vi "_PC_Daemon_AO&DO.vi"(7 "eng_mode":refnum<vi>, 8 "error in (no error)":errorcluster) -> (0 "error out":errorcluster)   [LabVIEW 2018]
uses:
  <vilib>/event_ctls.llb/eventvkey.ctl
  RTFunc/_PC_RTFunc_AccessExtAO.vi
  RTFunc/_PC_RTFunc_AccessExtDI.vi
  RTFunc/_PC_RTFunc_AccessExtDO.vi
  PublicSubVI/Class/QMH/QMH.lvclass
panel:
  in  "Tab Control":T1(tab)
  in  "AO.Apply":bool
  in  "AO 7":cluster{"Label":string, "y":dbl}
  in  "AO 6":cluster{"Label":string, "y":dbl}
  in  "AO 5":cluster{"Label":string, "y":dbl}
  in  "AO 4":cluster{"Label":string, "y":dbl}
  in  "AO 3":cluster{"Label":string, "y":dbl}
  in  "AO 2":cluster{"Label":string, "y":dbl}
  in  "AO 1":cluster{"Label":string, "y":dbl}
  in  "AO 0":cluster{"Label":string, "y":dbl}
  in  "DO 7":cluster{"Label":string, "Boolean":bool}
  in  "DO 6":cluster{"Label":string, "Boolean":bool}
  in  "DO 5":cluster{"Label":string, "Boolean":bool}
  in  "DO 4":cluster{"Label":string, "Boolean":bool}
  in  "DO 3":cluster{"Label":string, "Boolean":bool}
  in  "DO 2":cluster{"Label":string, "Boolean":bool}
  in  "DO 1":cluster{"Label":string, "Boolean":bool}
  in  "DO 0":cluster{"Label":string, "Boolean":bool}
  in  "DO.Apply":bool
  in  "DI 7":cluster{"Label":string, "Boolean":bool}
  in  "DI 6":cluster{"Label":string, "Boolean":bool}
  in  "DI 5":cluster{"Label":string, "Boolean":bool}
  in  "DI 4":cluster{"Label":string, "Boolean":bool}
  in  "DI 3":cluster{"Label":string, "Boolean":bool}
  in  "DI 2":cluster{"Label":string, "Boolean":bool}
  in  "DI 1":cluster{"Label":string, "Boolean":bool}
  in  "DI 0":cluster{"Label":string, "Boolean":bool}
  in  "DI.Apply":bool
  out "stop":bool
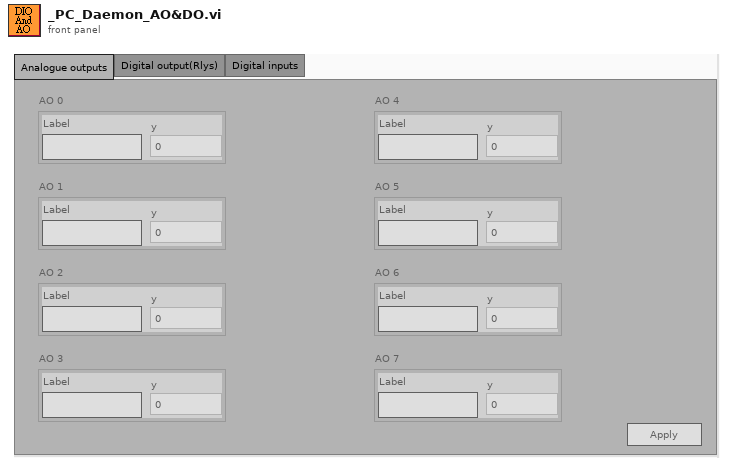
[diagram p1: front panel]
types:
  T1 = enum32{"Analogue outputs", "Digital output(Rlys)", "Digital inputs"}
  T2 = enum32{"Invalid", "Default", "Floating", "Floating/Auto-Hide", "Modal"}
  T3 = enum8{"Enabled", "Disabled", "Disabled and Grayed Out"}
  T4 = typedef "_ctl_RT_ExtAO.ctl" = cluster{"Label":string, "y":dbl}[]
  T5 = typedef "eventvkey.ctl" = enum16{"ASCII", "Enter", "Return", "Shift", "Ctrl", "Alt", "Cmd", "Opt", "Caps", "NumLock", "Clear", "Break", "Up", "Down", "Left", "Right", "Insert", "Delete", "Home", "End", "PageUp", "PageDown", "Escape", "Help", "Pause", "ScrollLock", "F1", "F2", "F3", "F4", "F5", "F6", "F7", "F8", "F9", "F10", "F11", "F12", "F13", "F14", "F15", "F16", "F17", "F18", "F19", "F20", "F21", "F22", "F23", "F24", "Play", "VolumeUp", "VolumeDown", "Mute", "Two Byte Char"}
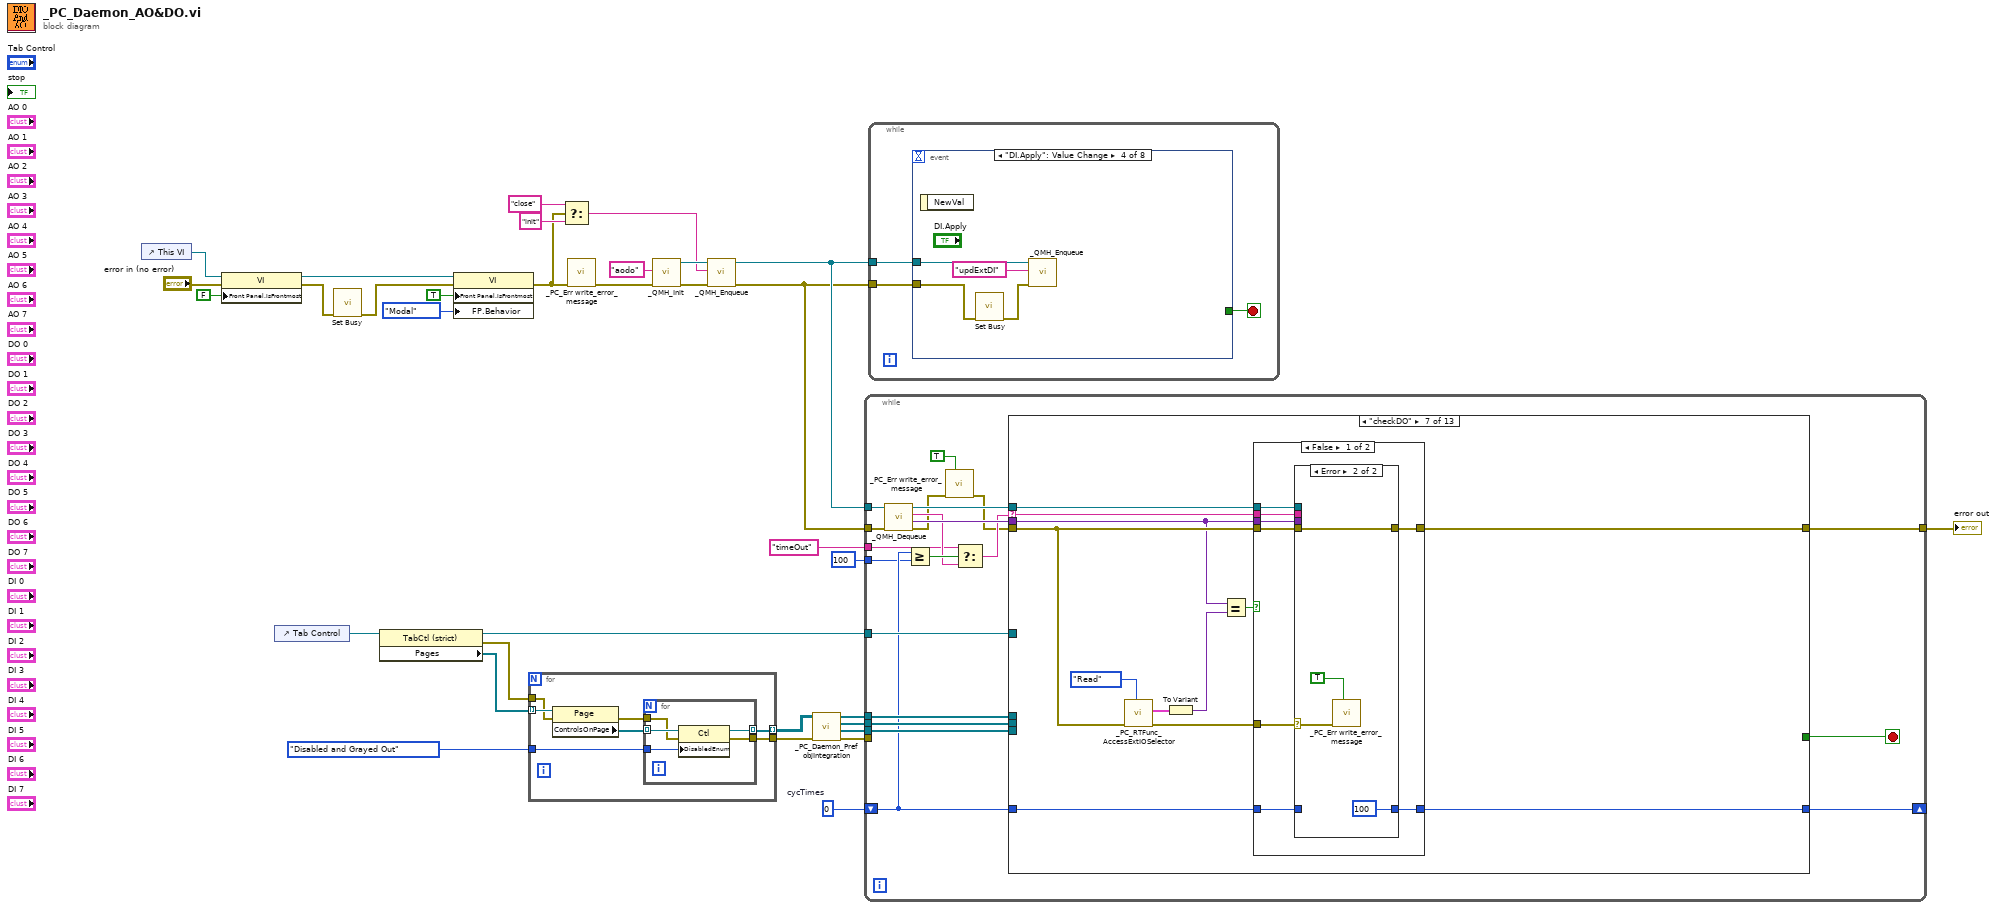
[diagram p0: block diagram]
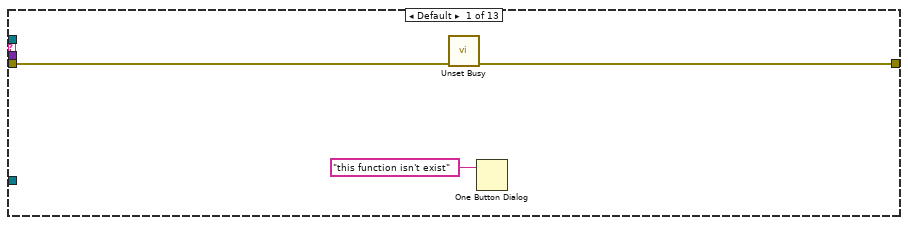
[diagram p2: hidden frame]
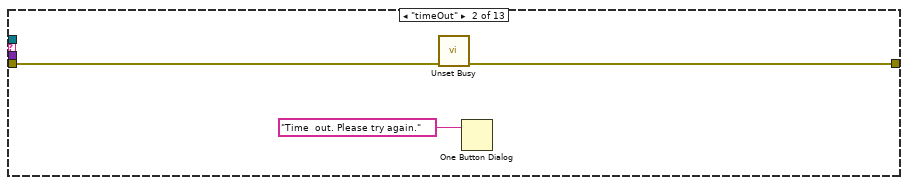
[diagram p3: hidden frame]
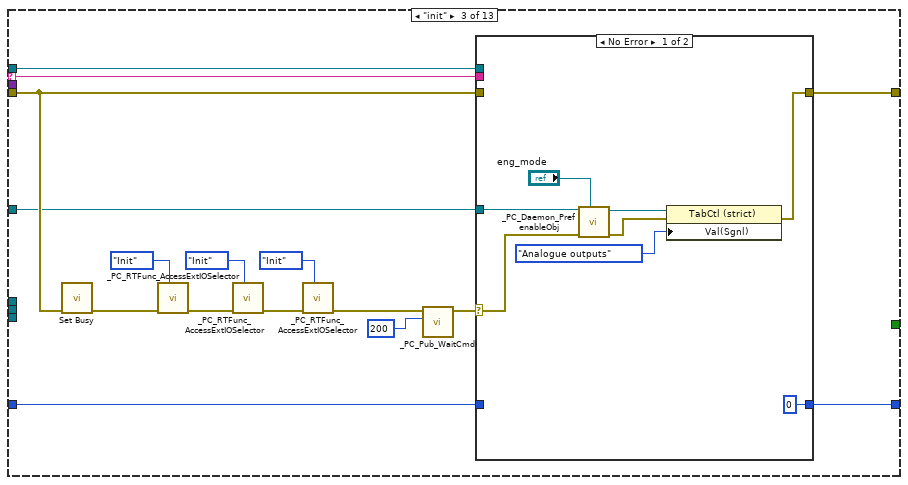
[diagram p4: hidden frame]
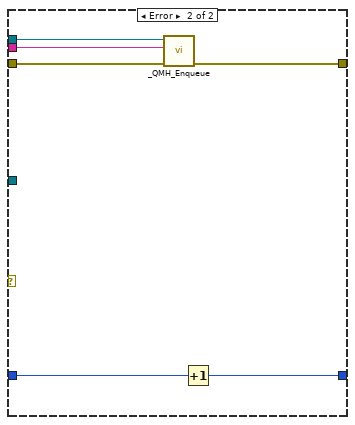
[diagram p5: hidden frame]
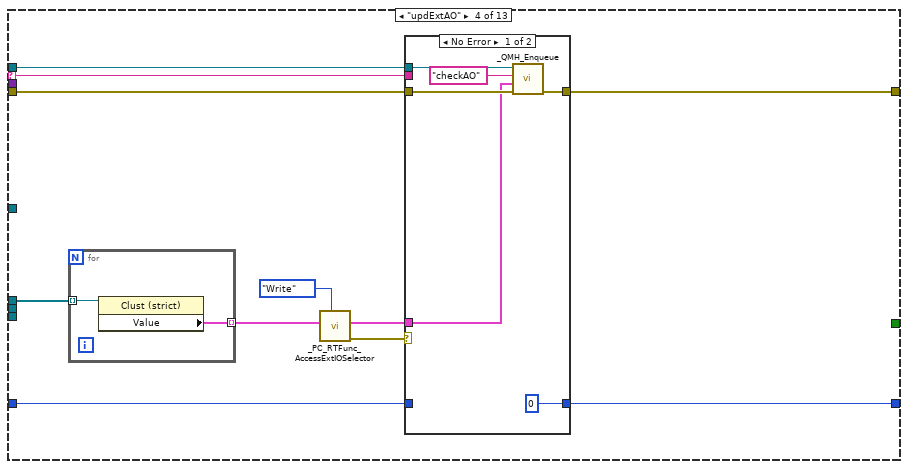
[diagram p6: hidden frame]
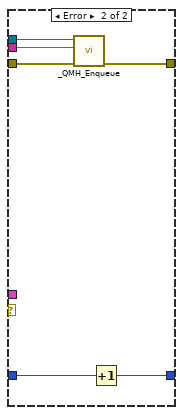
[diagram p7: hidden frame]
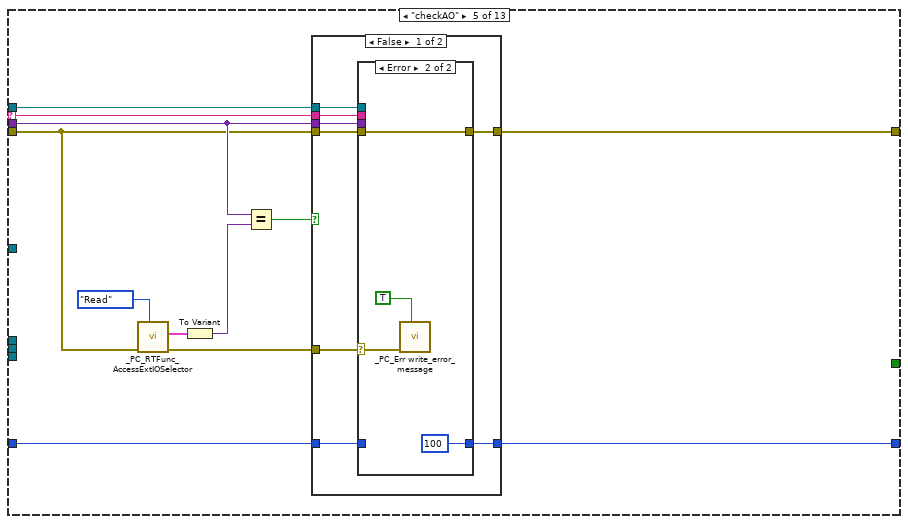
[diagram p8: hidden frame]
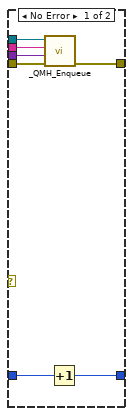
[diagram p9: hidden frame]
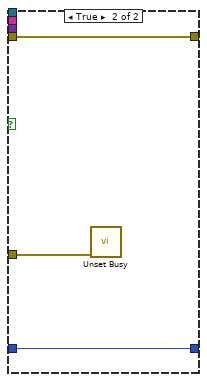
[diagram p10: hidden frame]
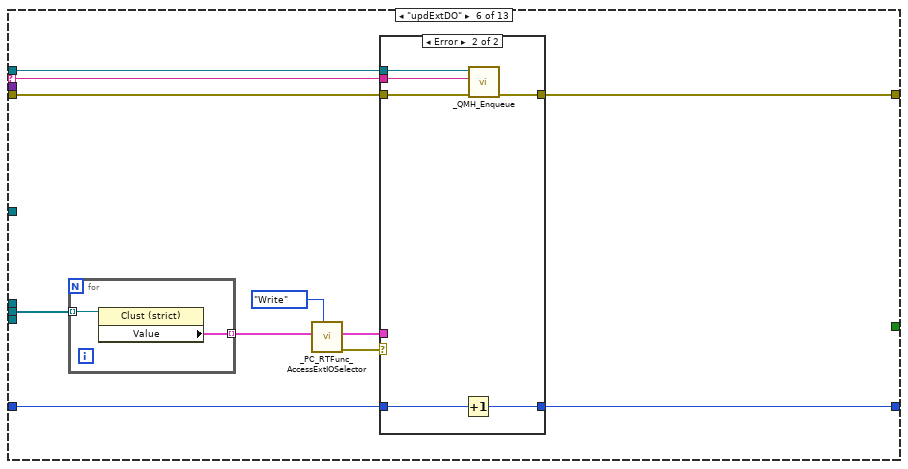
[diagram p11: hidden frame]
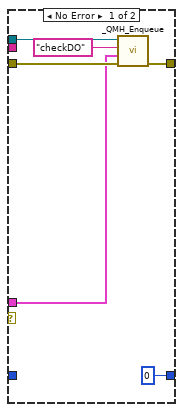
[diagram p12: hidden frame]
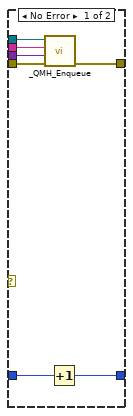
[diagram p13: hidden frame]
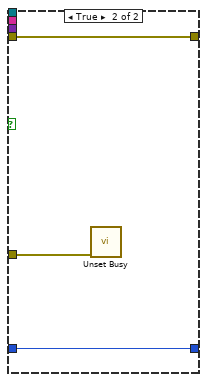
[diagram p14: hidden frame]
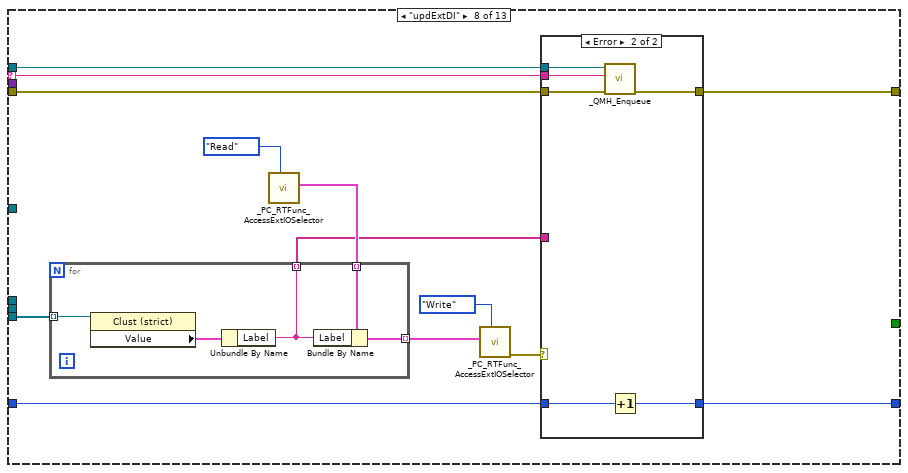
[diagram p15: hidden frame]
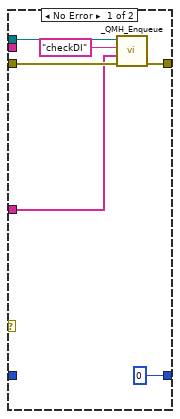
[diagram p16: hidden frame]
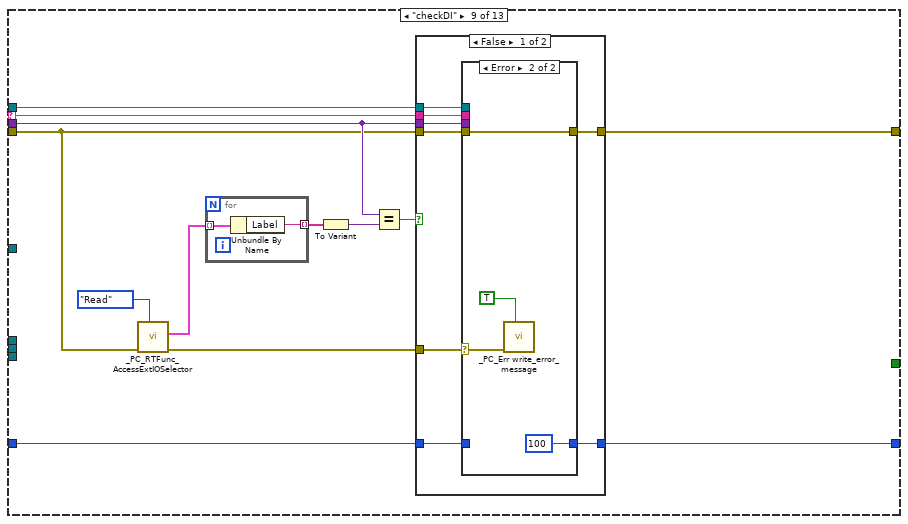
[diagram p17: hidden frame]
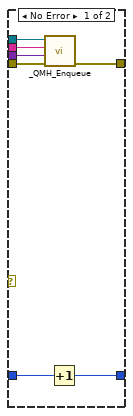
[diagram p18: hidden frame]
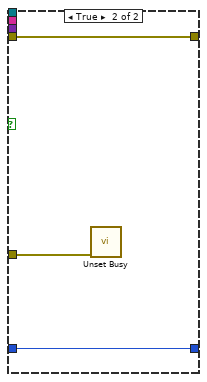
[diagram p19: hidden frame]
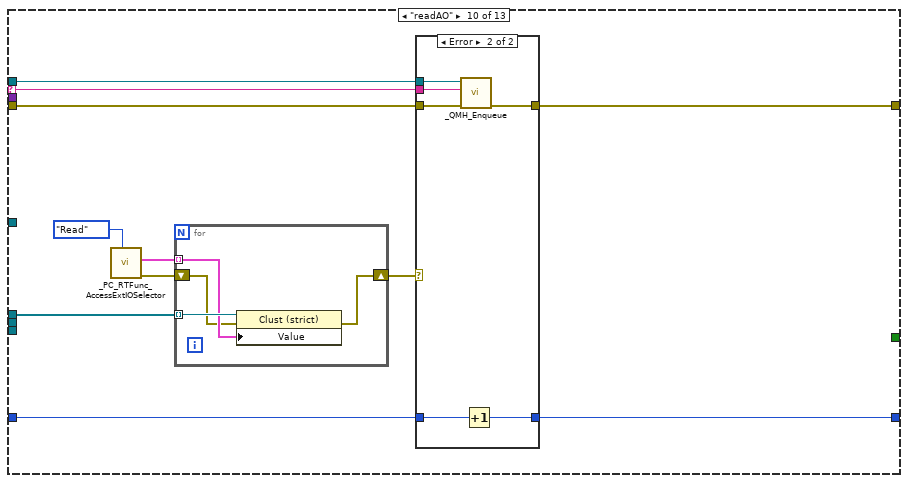
[diagram p20: hidden frame]
diagram:
  w3 = 0  # cycTimes
  n1 = control-ref of="This VI"() -> (w24:refnum<vi>)
  n2 = property class="VI"(reference=w24, error in="error in (no error)", "Front Panel.IsFrontmost"=FALSE) -> (reference out=w21:refnum<vi>, error out=w22:errorcluster)
  n3 = control-ref of="Tab Control"() -> (w33:refnum<vi>)
  n4 = call <vilib>:"Set Busy.vi"("error in (no error)"=w22) -> ("error out"=w20:errorcluster)  [unwired: 9 in, 1 out]
  n5 = property class="TabCtl (strict)"(reference=w33) -> (reference out=w5:refnum<vi>, error out=w32:errorcluster, "Pages"=w31:refnum<vi>[])  [unwired: 1 in]
  n6 = property class="VI"(reference=w21, error in=w20, "Front Panel.IsFrontmost"=TRUE ("Front Panel Window:Is Frontmost"), "FP.Behavior"=T2."Modal" ("Front Panel Window:Behavior")) -> (error out=w13:errorcluster)  [unwired: 1 out]
  n7 = for {
    tunnel: w31 -> [w40] mode=indexing
    tunnel: T3."Disabled and Grayed Out" ("Disabled") -> [w39]
    tunnel: [w37] -> w28
    tunnel: w32 -> [w35]
    tunnel: [w34] -> w29 mode=indexing
    n8 = property class="Page"(reference=w40, error in=w35) -> (error out=w36:errorcluster, "ControlsOnPage"=w38:refnum<vi>[])  [unwired: 1 out]
    n9 = for {
      tunnel: w38 -> [w45] mode=indexing
      tunnel: w39 -> [w44]
      tunnel: [w43] -> w37
      tunnel: w36 -> [w42]
      tunnel: [w41] -> w34 mode=indexing
      n10 = property class="Ctl"(reference=w45, error in=w42, "DisabledEnum"=w44) -> (reference out=w41:refnum<vi>, error out=w43:errorcluster)
    }
  }
  n11 = Select(t="close" ("name (unnamed)"), s=w13, f="init") -> (s? t:f=w15:string)
  n12 = call "_PC_Err write_error_message.vi"("error in"=w13) -> ("error out"=w12:errorcluster)  [unwired: 10 in]
  n13 = call "_QMH_Init.vi"("error in (no error)"=w12, "name (unnamed)"="aodo") -> ("error out"=w14:errorcluster, "QMH out"=w16:refnum<class "QMH.lvclass">)  [unwired: 8 in]
  n14 = call "_QMH_Enqueue.vi"("error in (no error)"=w14, "Msg"=w15, "QMH in"=w16) -> ("error out"=w10:errorcluster, "QMH out"=w11:refnum<class "QMH.lvclass">)  [unwired: 7 in]
  n15 = call "_PC_Daemon_Pref objIntegration.vi"("error in (no error)"=w28, "tabObjRefnum"=w29) -> ("error out"=w6:errorcluster, "DI"=w7:refnum<vi>[], "DO"=w8:refnum<vi>[], "AO"=w9:refnum<vi>[])  [unwired: 6 in]
  n16 = while {
    tunnel: w9 -> [w63]
    tunnel: w11 -> [w65]
    tunnel: w10 -> [w64]
    tunnel: w5 -> [w60]
    tunnel: w8 -> [w59]
    tunnel: w7 -> [w58]
    tunnel: w6 -> [_]
    tunnel: [w56] -> w4
    shift-right: [w55] -> _
    shift-left: w3 -> [w54]
    tunnel: 100 ("y") -> [w53]
    tunnel: "timeOut" ("t") -> [w49]
    stop <- w57 stop-if-true
    n17 = call "_QMH_Dequeue.vi"("error in (no error)"=w64, "QMH in"=w65) -> ("error out"=w47:errorcluster, "Data"=w61:variant, "Msg"=w51:string, "QMH out"=w62:refnum<class "QMH.lvclass">)  [unwired: 4 in, 2 out]
    n18 = Greater Or Equal?(x=w54, y=w53) -> (x >= y?=w52:bool)
    n19 = call "_PC_Err write_error_message.vi"("show msg( T )"=TRUE, "error in"=w47) -> ("error out"=w46:errorcluster)  [unwired: 9 in]
    n20 = Select(t=w49, s=w52, f=w51) -> (s? t:f=w50:string)
    n21 = case shown="\"checkDO\"" w50 {
      selector: w50 -> [_ _ w75 w107 w131 w166 w190 w228 w257 w291 w316 w340 _]
      tunnel: w63 -> [_ _ _ w106 _ _ _ _ _ w295 _ _ _]
      tunnel: w46 -> [w67 w70 w77 w108 w129 w167 w191 w229 w255 w290 w315 w339 w360]
      tunnel: w62 -> [_ _ w78 w109 w132 w168 w192 w230 w258 w292 w317 w341 w361]
      tunnel: w61 -> [_ _ _ _ w130 _ w189 _ w256 _ _ _ _]
      tunnel: w60 -> [_ _ w76 _ _ _ _ _ _ _ _ _ _]
      tunnel: w59 -> [_ _ _ _ _ w164 _ _ _ _ w318 _ _]
      tunnel: w58 -> [_ _ _ _ _ _ _ w226 _ _ _ w342 _]
      tunnel: [_ _ _ _ _ _ _ _ _ _ _ _ TRUE] -> w57
      tunnel: [w66 w69 w72 w102 w128 w161 w186 w220 w250 w287 w314 w335 w359] -> w56
      tunnel: w54 -> [_ _ w74 w104 w135 w163 w188 w222 w252 w289 w312 w337 _]
      tunnel: [_ _ w73 w103 w127 w162 w187 w221 w251 w288 w313 w336 _] -> w55
      frame Default {
        n22 = call <vilib>:"Unset Busy.vi"("error in (no error)"=w67) -> ("error out"=w66:errorcluster)  [unwired: 10 in]
        n23 = One Button Dialog(message="this function isn't exist") -> ()  [unwired: 1 in, 1 out]
      }
      frame "timeOut" {
        n24 = call <vilib>:"Unset Busy.vi"("error in (no error)"=w70) -> ("error out"=w69:errorcluster)  [unwired: 10 in]
        n25 = One Button Dialog(message="Time  out. Please try again.") -> ()  [unwired: 1 in, 1 out]
      }
      frame "init" {
        n26 = call <vilib>:"Set Busy.vi"("error in (no error)"=w77) -> ("error out"=w82:errorcluster)  [unwired: 9 in, 1 out]
        n27 = call-poly "_PC_RTFunc_AccessExtIOSelector.vi"("Function"=enum16{"Init", "Write", "Read"}."Init", "error in (no error)"=w82) -> ("error out"=w84:errorcluster)  [unwired: 8 in, 1 out]
        n28 = call-poly "_PC_RTFunc_AccessExtIOSelector.vi"("Function"=enum16{"Init", "Write", "Read"}."Init", "error in (no error)"=w84) -> ("error out"=w83:errorcluster)  [unwired: 8 in, 1 out]
        n29 = call-poly "_PC_RTFunc_AccessExtIOSelector.vi"("Function"=enum16{"Init", "Write", "Read"}."Init", "error in (no error)"=w83) -> ("error out"=w80:errorcluster)  [unwired: 8 in, 1 out]
        n30 = call "_PC_Pub_WaitCmd.vi"("milliseconds to wait"=u32 200, "error in (no error)"=w80) -> ("error out"=w79:errorcluster)  [unwired: 9 in]
        n31 = case shown="No Error" w79 {
          selector: w79 -> [w93 _]
          tunnel: w78 -> [_ w101]
          tunnel: w77 -> [_ w100]
          tunnel: w76 -> [w91 _]
          tunnel: w75 -> [_ w99]
          tunnel: w74 -> [_ w98]
          tunnel: [0 w97] -> w73
          tunnel: [w88 w96] -> w72
          frame No Error {
            n32 = call "_PC_Daemon_Pref enableObj.vi"("engModeStr"="eng_mode", "error in (no error)"=w93, "tabCtrlRefnum in"=w91) -> ("error out"=w92:errorcluster, "tabCtrlRefnum out"=w90:refnum<vi>)  [unwired: 7 in]
            n33 = property class="TabCtl (strict)"(reference=w90, error in=w92, "Val(Sgnl)"=T1."Analogue outputs" ("Value (Signaling)")) -> (error out=w88:errorcluster)  [unwired: 1 out]
          }
          frame Error {
            n34 = call "_QMH_Enqueue.vi"("error in (no error)"=w100, "Msg"=w99, "QMH in"=w101) -> ("error out"=w96:errorcluster)  [unwired: 7 in, 1 out]
            n35 = Increment(x=w98) -> (x+1=w97:i32)
          }
        }
      }
      frame "updExtAO" {
        n36 = for {
          tunnel: w106 -> [w126] mode=indexing
          tunnel: [w125] -> w105 mode=indexing
          n37 = property class="Clust (strict)"(reference=w126) -> ("Value"=w125:cluster{"Label":string, "y":dbl})  [unwired: 1 in, 2 out]
        }
        n38 = call-poly "_PC_RTFunc_AccessExtIOSelector.vi"("Function"=enum16{"Init", "Write", "Read"}."Write", "AnalogueOutput in"=w105) -> ("error out"=w111:errorcluster, "AnalogueOutput out"=w110:T4)  [unwired: 8 in]
        n39 = case shown="No Error" w111 {
          tunnel: w110 -> [w115 _]
          tunnel: w109 -> [w118 w124]
          tunnel: w108 -> [w117 w122]
          tunnel: w107 -> [_ w123]
          tunnel: w104 -> [_ w121]
          tunnel: [0 w120] -> w103
          tunnel: [w113 w119] -> w102
          frame No Error {
            n40 = call "_QMH_Enqueue.vi"("error in (no error)"=w117, "Data"=w115, "Msg"="checkAO", "QMH in"=w118) -> ("error out"=w113:errorcluster)  [unwired: 6 in, 1 out]
          }
          frame Error {
            n41 = call "_QMH_Enqueue.vi"("error in (no error)"=w122, "Msg"=w123, "QMH in"=w124) -> ("error out"=w119:errorcluster)  [unwired: 7 in, 1 out]
            n42 = Increment(x=w121) -> (x+1=w120:i32)
          }
        }
      }
      frame "checkAO" {
        n43 = call-poly "_PC_RTFunc_AccessExtIOSelector.vi"("Function"=enum16{"Init", "Write", "Read"}."Read", "error in (no error)"=w129) -> ("error out"=w134:errorcluster, "AnalogueOutput out"=w137:T4)  [unwired: 8 in]
        n44 = To Variant(anything=w137) -> (Variant=w136:variant)
        n45 = Equal?(x=w130, y=w136) -> (x = y?=w133:bool)
        n46 = case shown="False" w133 {
          tunnel: w134 -> [w144 w160]
          tunnel: w132 -> [w146 _]
          tunnel: w129 -> [w145 w158]
          tunnel: w131 -> [w143 _]
          tunnel: w130 -> [w142 _]
          tunnel: w135 -> [w141 w159]
          tunnel: [w140 w159] -> w127
          tunnel: [w139 w158] -> w128
          frame False {
            n47 = case shown="Error" w144 {
              selector: w144 -> [_ w156]
              tunnel: w146 -> [w153 _]
              tunnel: w145 -> [w150 w154]
              tunnel: w143 -> [w152 _]
              tunnel: w142 -> [w151 _]
              tunnel: w141 -> [w149 _]
              tunnel: [w148 100] -> w140
              tunnel: [w147 w154] -> w139
              frame No Error {
                n48 = call "_QMH_Enqueue.vi"("error in (no error)"=w150, "Data"=w151, "Msg"=w152, "QMH in"=w153) -> ("error out"=w147:errorcluster)  [unwired: 6 in, 1 out]
                n49 = Increment(x=w149) -> (x+1=w148:i32)
              }
              frame Error {
                n50 = call "_PC_Err write_error_message.vi"("show msg( T )"=TRUE, "error in"=w156) -> ()  [unwired: 9 in, 1 out]
              }
            }
          }
          frame True {
            n51 = call <vilib>:"Unset Busy.vi"("error in (no error)"=w160) -> ()  [unwired: 10 in, 1 out]
          }
        }
      }
      frame "updExtDO" {
        n52 = for {
          tunnel: w164 -> [w185] mode=indexing
          tunnel: [w184] -> w165 mode=indexing
          n53 = property class="Clust (strict)"(reference=w185) -> ("Value"=w184:cluster{"Label":string, "Boolean":bool})  [unwired: 1 in, 2 out]
        }
        n54 = call-poly "_PC_RTFunc_AccessExtIOSelector.vi"("Function"=enum16{"Init", "Write", "Read"}."Write", "DO in"=w165) -> ("error out"=w170:errorcluster, "DO out"=w169:cluster{"Label":string, "Boolean":bool}[])  [unwired: 8 in]
        n55 = case shown="Error" w170 {
          tunnel: w169 -> [w174 _]
          tunnel: w168 -> [w177 w183]
          tunnel: w167 -> [w176 w178]
          tunnel: w166 -> [_ w182]
          tunnel: w163 -> [_ w179]
          tunnel: [0 w181] -> w162
          tunnel: [w172 w180] -> w161
          frame No Error {
            n56 = call "_QMH_Enqueue.vi"("error in (no error)"=w176, "Data"=w174, "Msg"="checkDO", "QMH in"=w177) -> ("error out"=w172:errorcluster)  [unwired: 6 in, 1 out]
          }
          frame Error {
            n57 = Increment(x=w179) -> (x+1=w181:i32)
            n58 = call "_QMH_Enqueue.vi"("error in (no error)"=w178, "Msg"=w182, "QMH in"=w183) -> ("error out"=w180:errorcluster)  [unwired: 7 in, 1 out]
          }
        }
      }
      frame "checkDO" {
        n59 = call-poly "_PC_RTFunc_AccessExtIOSelector.vi"("Function"=enum16{"Init", "Write", "Read"}."Read", "error in (no error)"=w191) -> ("error out"=w193:errorcluster, "DO out"=w196:cluster{"Label":string, "Boolean":bool}[])  [unwired: 8 in]
        n60 = To Variant(anything=w196) -> (Variant=w195:variant)
        n61 = Equal?(x=w189, y=w195) -> (x = y?=w194:bool)
        n62 = case shown="False" w194 {
          tunnel: w193 -> [w203 w219]
          tunnel: w192 -> [w205 _]
          tunnel: w191 -> [w204 w217]
          tunnel: w190 -> [w202 _]
          tunnel: w189 -> [w201 _]
          tunnel: w188 -> [w200 w218]
          tunnel: [w199 w218] -> w187
          tunnel: [w198 w217] -> w186
          frame False {
            n63 = case shown="Error" w203 {
              selector: w203 -> [_ w215]
              tunnel: w205 -> [w212 _]
              tunnel: w204 -> [w209 w213]
              tunnel: w202 -> [w211 _]
              tunnel: w201 -> [w210 _]
              tunnel: w200 -> [w208 _]
              tunnel: [w207 100] -> w199
              tunnel: [w206 w213] -> w198
              frame No Error {
                n64 = call "_QMH_Enqueue.vi"("error in (no error)"=w209, "Data"=w210, "Msg"=w211, "QMH in"=w212) -> ("error out"=w206:errorcluster)  [unwired: 6 in, 1 out]
                n65 = Increment(x=w208) -> (x+1=w207:i32)
              }
              frame Error {
                n66 = call "_PC_Err write_error_message.vi"("show msg( T )"=TRUE, "error in"=w215) -> ()  [unwired: 9 in, 1 out]
              }
            }
          }
          frame True {
            n67 = call <vilib>:"Unset Busy.vi"("error in (no error)"=w219) -> ()  [unwired: 10 in, 1 out]
          }
        }
      }
      frame "updExtDI" {
        n68 = call-poly "_PC_RTFunc_AccessExtIOSelector.vi"("Function"=enum16{"Init", "Write", "Read"}."Read") -> ("DI out"=w224:cluster{"Label":string, "Boolean":bool}[])  [unwired: 9 in, 1 out]
        n69 = for {
          tunnel: w226 -> [w249] mode=indexing
          tunnel: [w245] -> w227 mode=indexing
          tunnel: w224 -> [w247] mode=indexing
          tunnel: [w246] -> w223 mode=indexing
          n70 = property class="Clust (strict)"(reference=w249) -> ("Value"=w248:cluster{"Label":string, "Boolean":bool})  [unwired: 1 in, 2 out]
          n71 = Unbundle By Name(w248) -> ("Label"=w246:string)
          n72 = Bundle By Name(cluster=w247, "Label"=w246) -> (w245:cluster{"Label":string, "Boolean":bool})
        }
        n73 = call-poly "_PC_RTFunc_AccessExtIOSelector.vi"("Function"=enum16{"Init", "Write", "Read"}."Write", "DI in"=w227) -> ("error out"=w231:errorcluster)  [unwired: 8 in, 1 out]
        n74 = case shown="Error" w231 {
          tunnel: w230 -> [w238 w244]
          tunnel: w229 -> [w237 w242]
          tunnel: w228 -> [_ w243]
          tunnel: w223 -> [w235 _]
          tunnel: w222 -> [_ w241]
          tunnel: [0 w240] -> w221
          tunnel: [w233 w239] -> w220
          frame No Error {
            n75 = call "_QMH_Enqueue.vi"("error in (no error)"=w237, "Data"=w235, "Msg"="checkDI", "QMH in"=w238) -> ("error out"=w233:errorcluster)  [unwired: 6 in, 1 out]
          }
          frame Error {
            n76 = call "_QMH_Enqueue.vi"("error in (no error)"=w242, "Msg"=w243, "QMH in"=w244) -> ("error out"=w239:errorcluster)  [unwired: 7 in, 1 out]
            n77 = Increment(x=w241) -> (x+1=w240:i32)
          }
        }
      }
      frame "checkDI" {
        n78 = call-poly "_PC_RTFunc_AccessExtIOSelector.vi"("Function"=enum16{"Init", "Write", "Read"}."Read", "error in (no error)"=w255) -> ("error out"=w253:errorcluster, "DI out"=w260:cluster{"Label":string, "Boolean":bool}[])  [unwired: 8 in]
        n79 = for {
          tunnel: w260 -> [w286] mode=indexing
          tunnel: [w285] -> w259 mode=indexing
          n80 = Unbundle By Name(w286) -> ("Label"=w285:string)
        }
        n81 = To Variant(anything=w259) -> (Variant=w261:variant)
        n82 = Equal?(x=w256, y=w261) -> (x = y?=w254:bool)
        n83 = case shown="False" w254 {
          tunnel: w253 -> [w268 w284]
          tunnel: w258 -> [w270 _]
          tunnel: w255 -> [w269 w282]
          tunnel: w257 -> [w267 _]
          tunnel: w256 -> [w266 _]
          tunnel: w252 -> [w265 w283]
          tunnel: [w264 w283] -> w251
          tunnel: [w263 w282] -> w250
          frame False {
            n84 = case shown="Error" w268 {
              selector: w268 -> [_ w280]
              tunnel: w270 -> [w277 _]
              tunnel: w269 -> [w274 w278]
              tunnel: w267 -> [w276 _]
              tunnel: w266 -> [w275 _]
              tunnel: w265 -> [w273 _]
              tunnel: [w272 100] -> w264
              tunnel: [w271 w278] -> w263
              frame No Error {
                n85 = call "_QMH_Enqueue.vi"("error in (no error)"=w274, "Data"=w275, "Msg"=w276, "QMH in"=w277) -> ("error out"=w271:errorcluster)  [unwired: 6 in, 1 out]
                n86 = Increment(x=w273) -> (x+1=w272:i32)
              }
              frame Error {
                n87 = call "_PC_Err write_error_message.vi"("show msg( T )"=TRUE, "error in"=w280) -> ()  [unwired: 9 in, 1 out]
              }
            }
          }
          frame True {
            n88 = call <vilib>:"Unset Busy.vi"("error in (no error)"=w284) -> ()  [unwired: 10 in, 1 out]
          }
        }
      }
      frame "readAO" {
        n89 = call-poly "_PC_RTFunc_AccessExtIOSelector.vi"("Function"=enum16{"Init", "Write", "Read"}."Read") -> ("error out"=w294:errorcluster, "AnalogueOutput out"=w296:T4)  [unwired: 9 in]
        n90 = for {
          tunnel: w296 -> [w309] mode=indexing
          tunnel: w295 -> [w310] mode=indexing
          shift-right: [w307] -> w293
          shift-left: w294 -> [w308]
          n91 = property class="Clust (strict)"(reference=w310, error in=w308, "Value"=w309) -> (error out=w307:errorcluster)  [unwired: 1 out]
        }
        n92 = case shown="Error" w293 {
          selector: w293 -> [w300 _]
          tunnel: w292 -> [_ w306]
          tunnel: w291 -> [_ w305]
          tunnel: w290 -> [w298 w304]
          tunnel: w289 -> [w299 w303]
          tunnel: [w299 w302] -> w288
          tunnel: [w298 w301] -> w287
          frame No Error {
            n93 = call <vilib>:"Unset Busy.vi"("error in (no error)"=w300) -> ()  [unwired: 10 in, 1 out]
          }
          frame Error {
            n94 = call "_QMH_Enqueue.vi"("error in (no error)"=w304, "Msg"=w305, "QMH in"=w306) -> ("error out"=w301:errorcluster)  [unwired: 7 in, 1 out]
            n95 = Increment(x=w303) -> (x+1=w302:i32)
          }
        }
      }
      frame "readDO" {
        n96 = call-poly "_PC_RTFunc_AccessExtIOSelector.vi"("Function"=enum16{"Init", "Write", "Read"}."Read") -> ("error out"=w319:errorcluster, "DO out"=w320:cluster{"Label":string, "Boolean":bool}[])  [unwired: 9 in]
        n97 = for {
          tunnel: w320 -> [w333] mode=indexing
          tunnel: w318 -> [w334] mode=indexing
          shift-right: [w331] -> w311
          shift-left: w319 -> [w332]
          n98 = property class="Clust (strict)"(reference=w334, error in=w332, "Value"=w333) -> (error out=w331:errorcluster)  [unwired: 1 out]
        }
        n99 = case shown="Error" w311 {
          selector: w311 -> [w324 _]
          tunnel: w317 -> [_ w330]
          tunnel: w316 -> [_ w329]
          tunnel: w315 -> [w322 w328]
          tunnel: w312 -> [w323 w327]
          tunnel: [w323 w326] -> w313
          tunnel: [w322 w325] -> w314
          frame No Error {
            n100 = call <vilib>:"Unset Busy.vi"("error in (no error)"=w324) -> ()  [unwired: 10 in, 1 out]
          }
          frame Error {
            n101 = call "_QMH_Enqueue.vi"("error in (no error)"=w328, "Msg"=w329, "QMH in"=w330) -> ("error out"=w325:errorcluster)  [unwired: 7 in, 1 out]
            n102 = Increment(x=w327) -> (x+1=w326:i32)
          }
        }
      }
      frame "readDI" {
        n103 = call-poly "_PC_RTFunc_AccessExtIOSelector.vi"("Function"=enum16{"Init", "Write", "Read"}."Read") -> ("error out"=w343:errorcluster, "DI out"=w344:cluster{"Label":string, "Boolean":bool}[])  [unwired: 9 in]
        n104 = for {
          tunnel: w344 -> [w357] mode=indexing
          tunnel: w342 -> [w356] mode=indexing
          shift-right: [w358] -> w338
          shift-left: w343 -> [w355]
          n105 = property class="Clust (strict)"(reference=w356, error in=w355, "Value"=w357) -> (error out=w358:errorcluster)  [unwired: 1 out]
        }
        n106 = case shown="Error" w338 {
          selector: w338 -> [w348 _]
          tunnel: w341 -> [_ w354]
          tunnel: w340 -> [_ w353]
          tunnel: w339 -> [w346 w352]
          tunnel: w337 -> [w347 w351]
          tunnel: [w347 w350] -> w336
          tunnel: [w346 w349] -> w335
          frame No Error {
            n107 = call <vilib>:"Unset Busy.vi"("error in (no error)"=w348) -> ()  [unwired: 10 in, 1 out]
          }
          frame Error {
            n108 = call "_QMH_Enqueue.vi"("error in (no error)"=w352, "Msg"=w353, "QMH in"=w354) -> ("error out"=w349:errorcluster)  [unwired: 7 in, 1 out]
            n109 = Increment(x=w351) -> (x+1=w350:i32)
          }
        }
      }
      frame "close" {
        n110 = call "_QMH_Close.vi"("error in (no error)"=w360, "QMH in"=w361) -> ("error out"=w359:errorcluster)  [unwired: 9 in]
        n111 = control-ref of="stop"() -> (w363:refnum<vi>)
        n112 = property class="Bool (strict)"(reference=w363, "Val(Sgnl)"=TRUE ("Value (Signaling)")) -> ()  [unwired: 1 in, 2 out]
      }
    }
  }
  "error out" <- w4
  n113 = while {
    tunnel: w11 -> [w367]
    tunnel: w10 -> [w366]
    stop <- w365 stop-if-true
    n114 = event shown="[3] \"DI.Apply\": Value Change" {
      selector: _ -> [_ _ _ _ _ _ _ _]
      dyn-events: _ -> [_ _ _ _ _ _ _ _]
      timeout: _ -> [_ _ _ _ _ _ _ _]
      tunnel: w367 -> [_ w370 w374 w378 w381 w399 w408 _]
      tunnel: w366 -> [_ w369 w373 w377 w380 w398 w405 _]
      tunnel: [_ _ _ _ _ _ _ w409] -> w365
      event Timeout {
        n115 = event-data() -> ()  [unwired: 1 in, 1 out]
      }
      event "AO.Apply": Value Change {
        n116 = event-data() -> ()  [unwired: 1 in, 1 out]
        n117 = call <vilib>:"Set Busy.vi"("error in (no error)"=w369) -> ("error out"=w368:errorcluster)  [unwired: 9 in, 1 out]
        n118 = call "_QMH_Enqueue.vi"("error in (no error)"=w368, "Msg"="updExtAO", "QMH in"=w370) -> ()  [unwired: 7 in, 2 out]
      }
      event "DO.Apply": Value Change {
        n119 = event-data() -> ()  [unwired: 1 in, 1 out]
        n120 = call <vilib>:"Set Busy.vi"("error in (no error)"=w373) -> ("error out"=w372:errorcluster)  [unwired: 9 in, 1 out]
        n121 = call "_QMH_Enqueue.vi"("error in (no error)"=w372, "Msg"="updExtDO", "QMH in"=w374) -> ()  [unwired: 7 in, 2 out]
      }
      event "DI.Apply": Value Change {
        n122 = event-data() -> ()  [unwired: 1 in, 1 out]
        n123 = call <vilib>:"Set Busy.vi"("error in (no error)"=w377) -> ("error out"=w376:errorcluster)  [unwired: 9 in, 1 out]
        n124 = call "_QMH_Enqueue.vi"("error in (no error)"=w376, "Msg"="updExtDI", "QMH in"=w378) -> ()  [unwired: 7 in, 2 out]
      }
      event "Tab Control": Value Change {
        n125 = event-data() -> ("NewVal"=w382:T1)  [unwired: 1 in]
        n126 = case shown="\"Digital inputs\"" w382 {
          tunnel: w381 -> [_ w385 w389 w393]
          tunnel: w380 -> [_ w384 w388 w392]
          frame Default {
          }
          frame "Digital inputs" {
            n127 = call <vilib>:"Set Busy.vi"("error in (no error)"=w384) -> ("error out"=w383:errorcluster)  [unwired: 9 in, 1 out]
            n128 = call "_QMH_Enqueue.vi"("error in (no error)"=w383, "Msg"="readDI", "QMH in"=w385) -> ()  [unwired: 7 in, 2 out]
          }
          frame "Digital output(Rlys)" {
            n129 = call <vilib>:"Set Busy.vi"("error in (no error)"=w388) -> ("error out"=w387:errorcluster)  [unwired: 9 in, 1 out]
            n130 = call "_QMH_Enqueue.vi"("error in (no error)"=w387, "Msg"="readDO", "QMH in"=w389) -> ()  [unwired: 7 in, 2 out]
          }
          frame "Analogue outputs" {
            n131 = call <vilib>:"Set Busy.vi"("error in (no error)"=w392) -> ("error out"=w391:errorcluster)  [unwired: 9 in, 1 out]
            n132 = call "_QMH_Enqueue.vi"("error in (no error)"=w391, "Msg"="readAO", "QMH in"=w393) -> ()  [unwired: 7 in, 2 out]
          }
        }
      }
      event Key Down? {
        n133 = event-data() -> ("VKey"=w397:T5)  [unwired: 1 in]
        n134 = Equal?(x=w397, y=eventvkey."Escape") -> (x = y?=w395:bool)
        n135 = case shown="True" w395 {
          tunnel: w399 -> [_ w403]
          tunnel: w398 -> [_ w401]
          frame False {
          }
          frame True {
            n136 = call <vilib>:"Set Busy.vi"("error in (no error)"=w401) -> ("error out"=w400:errorcluster)  [unwired: 9 in, 1 out]
            n137 = call "_QMH_Enqueue.vi"("error in (no error)"=w400, "Msg"="close", "QMH in"=w403) -> ()  [unwired: 7 in, 2 out]
          }
        }
        n138 = event-data("Discard?"=w395) -> ()  [unwired: 1 in, 1 out]
      }
      event Panel Close? {
        n139 = event-data() -> ()  [unwired: 1 in, 1 out]
        n140 = call <vilib>:"Set Busy.vi"("error in (no error)"=w405) -> ("error out"=w404:errorcluster)  [unwired: 9 in, 1 out]
        n141 = call "_QMH_Enqueue.vi"("error in (no error)"=w404, "Msg"="close", "QMH in"=w408) -> ()  [unwired: 7 in, 2 out]
        n142 = event-data("Discard?"=TRUE) -> ()  [unwired: 1 in, 1 out]
      }
      event "stop": Value Change {
        n143 = event-data() -> ("NewVal"=w409:bool)  [unwired: 1 in]
      }
    }
  }
